vi "Send Data.vi"(9 "Array 2":bool[](array[boolean]), 10 "Array":bool[](array[boolean]), 11 "VISA Input":refnum<visa-resource-name>) -> (3 "VISA Output":refnum<visa-resource-name>)   [LabVIEW 2009]
panel:
  out "String":string
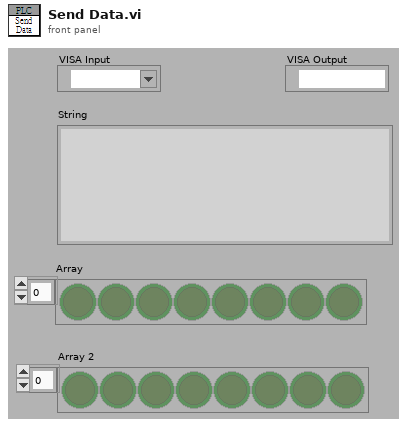
[diagram p1: front panel]
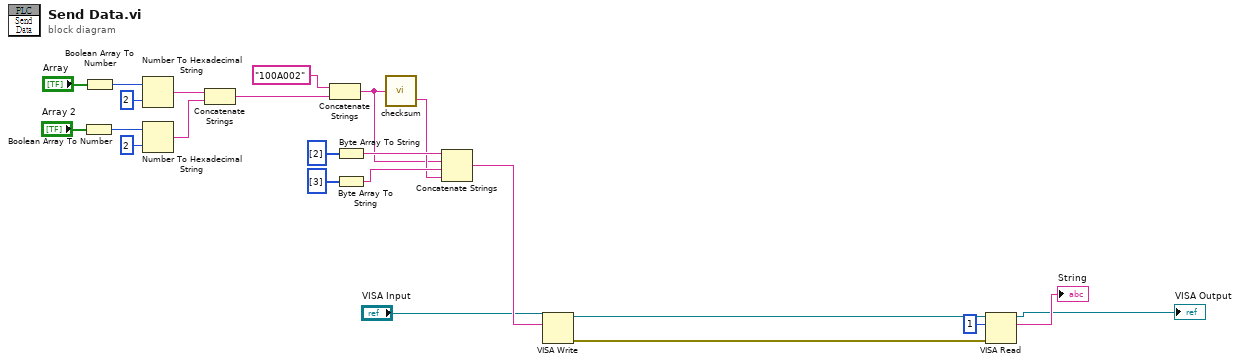
[diagram p0: block diagram]
diagram:
  n1 = Boolean Array To Number(Boolean array="Array 2") -> (number=w18:u32)
  n2 = Boolean Array To Number(Boolean array="Array") -> (number=w21:u32)
  n3 = Number To Hexadecimal String(1:i16 2 ("width (-)"), 2:w21) -> (0:w10:string)
  n4 = Number To Hexadecimal String(1:i16 2 ("width (-)"), 2:w18) -> (0:w9:string)
  n5 = Concatenate Strings(w10, w9) -> (w7:string)
  n6 = Concatenate Strings("100A002", w7) -> (w6:string)
  n7 = Byte Array To String(unsigned byte array=u8[] [2]) -> (string=w15:string)
  n8 = Byte Array To String(unsigned byte array=u8[] [3]) -> (string=w14:string)
  n9 = call "checksum.vi"("Data"=w6) -> ("Check Sum"=w13:string)  [unwired: 2 in, 1 out]
  n10 = Concatenate Strings(w15, w6, w14, w13) -> (w12:string)
  n11 = VISA Write(VISA resource name="VISA Input", write buffer=w12) -> (VISA resource name out=w3:refnum<visa-resource-name>, error out=w2:errorcluster)  [unwired: 1 in, 1 out]
  n12 = VISA Read(VISA resource name=w3, byte count=u32 1, error in (no error)=w2) -> (VISA resource name out=→"VISA Output":refnum<visa-resource-name>, read buffer=→"String":string)  [unwired: 2 out]
